vi "Configure Scale Over.vi"(0 "VISA resource name":refnum<visa-resource-name>, 5 "Scale Over (0: Free)":u16(ring) items=["Free", "Over"], 11 "error in (no error)":errorcluster) -> (4 "VISA resource name out":refnum<visa-resource-name>, 15 "error out":errorcluster)   [LabVIEW 2020, in "Yokogawa GX Series.lvlib"]
doc: "Sets method at scale over.\n\nCommand: SScaleOver"
uses:
  <instrlib>/Yokogawa GX Series/Yokogawa GX Series.lvlib
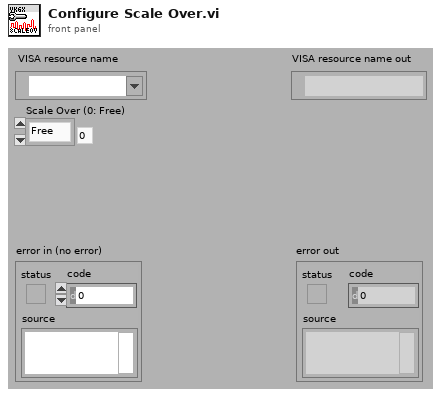
[diagram p1: front panel]
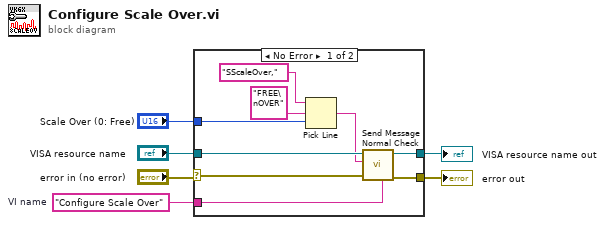
[diagram p0: block diagram]
diagram:
  w6 = "Configure Scale Over"  # VI name
  n1 = case shown="No Error" "error in (no error)" {
    selector: "error in (no error)" -> [w7 w17]
    tunnel: w6 -> [w15 _]
    tunnel: [w14 w16] -> w5
    tunnel: "VISA resource name" -> [w13 w16]
    tunnel: "Scale Over (0: Free)" -> [w12 _]
    tunnel: [w8 w17] -> w2
    frame No Error {
      n2 = Pick Line(string ("")="SScaleOver,", multi-line string="FREE\nOVER", line index=w12) -> (output string=w11:string)
      n3 = call <instrlib>:"Send Message Normal Check.vi"("Source (\"\")"=w15, "error in (no error)"=w7, "Send Message (\"\")"=w11, "VISA resource name"=w13) -> ("error out"=w8:errorcluster, "VISA resource name out"=w14:refnum<visa-resource-name>)  [unwired: 2 in, 4 out]
    }
    frame Error {
    }
  }
  "error out" <- w2
  "VISA resource name out" <- w5
